vi "Connect.vi"(8 "error in (no error)":errorcluster, 10 "Timeout":i32=2000, 11 "ClientBase in":refnum<class "ClientBase.lvclass">) -> (0 "error out":errorcluster, 3 "ClientBase out":refnum<class "ClientBase.lvclass">)   [LabVIEW 2020, in "ClientBaseLib.lvlib" / "ClientBase.lvclass"]
uses:
  ClientBase.lvclass
  ClientBase.lvclass/ClientBase.ctl
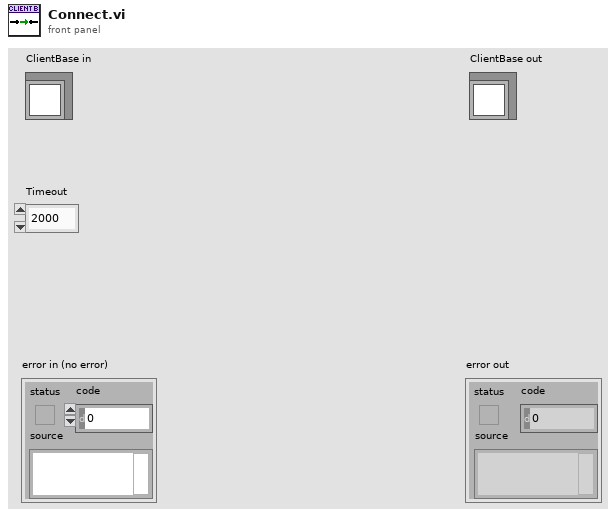
[diagram p1: front panel]
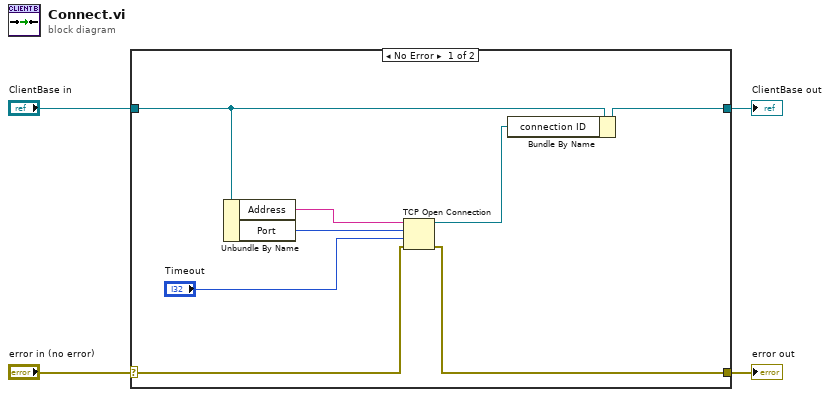
[diagram p0: block diagram]
diagram:
  n1 = case shown="No Error" "error in (no error)" {
    selector: "error in (no error)" -> [w8 w14]
    tunnel: [w7 w14] -> w3
    tunnel: [w6 w13] -> w1
    tunnel: "ClientBase in" -> [w12 w13]
    frame No Error {
      n2 = Unbundle By Name(w12) -> ("Address"=w11:string, "Port"=w10:u16)
      n3 = TCP Open Connection(address=w11, remote port or service name=w10, timeout ms (60000)="Timeout", error in (no error)=w8) -> (connection ID=w5:refnum<k5>, error out=w7:errorcluster)  [unwired: 1 in]
      n4 = Bundle By Name(cluster=w12, "connection ID"=w5) -> (w6:refnum<class "ClientBase.lvclass">)
    }
    frame Error {
    }
  }
  "error out" <- w3
  "ClientBase out" <- w1
